vi "N-Wave Memory Generator.vi"(11 "n":i32=1) -> (0 "FXP Init Data Out":fxp<+/-,12,12>[](array[numeric]), 3 "Init Data Out":i64[](array[numeric]))   [LabVIEW 2014]
uses:
  <vilib>/Analysis/NI_AALPro.lvlib
  <vilib>/Analysis/NI_AALBase.lvlib
panel:
  out "size(s)":i32
  out "Init Data Out Graph":i64[](graph)
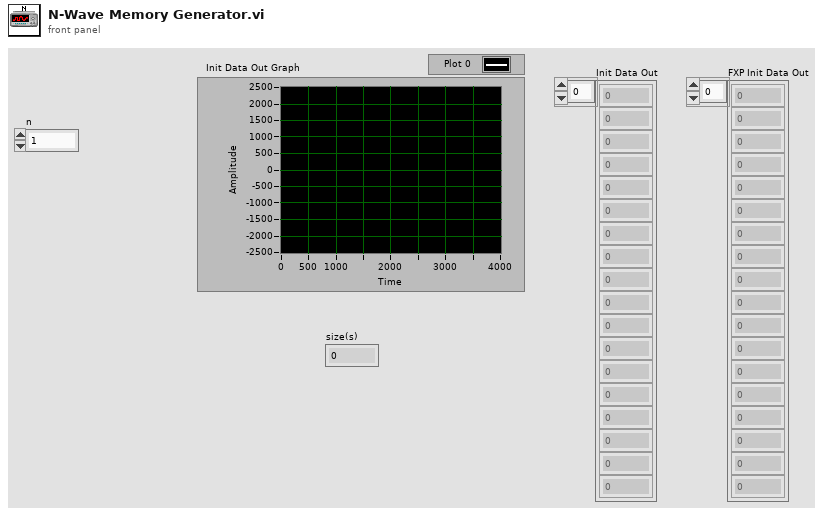
[diagram p1: front panel]
types:
  T1 = enum16{"sine", "cosine", "triangle", "square", "sawtooth", "increasing ramp", "decreasing ramp"}
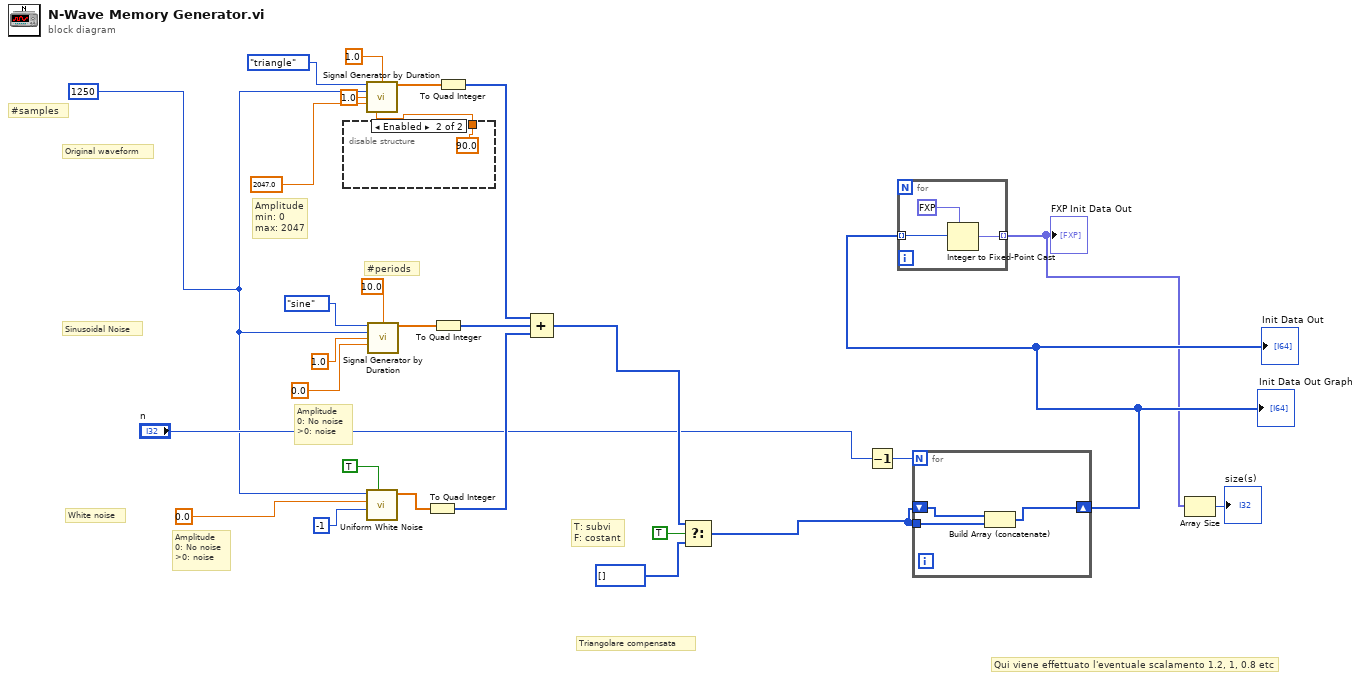
[diagram p0: block diagram]
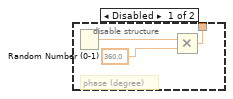
[diagram p2: hidden frame]
diagram:
  w5 = 1250 ("# of samples")
  # "Triangolare compensata"
  # "Qui viene effettuato l'eventuale scalamento 1.2, 1, 0.8 etc"
  # "T: subvi\nF: costant"
  # "Amplitude\n0: No noise\n>0: noise"
  # "Original waveform"
  # "Sinusoidal Noise"
  # "White noise"
  # "#periods"
  # "Amplitude\n0: No noise\n>0: noise"
  # "Amplitude\nmin: 0\nmax: 2047"
  # "#samples"
  n1 = disable-structure shown="Enabled" {
    disable-tunnel: [w29 90.0 ("phase in")] -> w14
    frame Disabled {
      # "phase (degree)"
      n2 = Random Number (0-1)() -> (number: 0 to 1=w30:dbl)
      n3 = Multiply(x=w30, y=360.0) -> (x*y=w29:dbl)
    }
    frame Enabled {
    }
  }
  n4 = call <vilib>:"Signal Generator by Duration.vi"("signal type"=T1."triangle", "duration"=1.0, "# of samples"=w5, "frequency"=1.0, "amplitude"=2047.0, "phase in"=w14) -> ("signal"=w16:dbl[])  [unwired: 6 in, 3 out]
  n5 = call <vilib>:"Uniform White Noise.vi"("initialize?"=TRUE, "seed"=-1, "amplitude"=0.0, "samples"=w5) -> ("uniform white noise"=w15:dbl[])  [unwired: 6 in, 1 out]
  n6 = call <vilib>:"Signal Generator by Duration.vi"("signal type"=T1."sine", "duration"=10.0, "# of samples"=w5, "frequency"=1.0, "amplitude"=0.0) -> ("signal"=w27:dbl[])  [unwired: 7 in, 3 out]
  n7 = To Quad Integer(1:w15) -> (0:w20:i64[])
  n8 = To Quad Integer(1:w27) -> (0:w22:i64[])
  n9 = To Quad Integer(1:w16) -> (0:w6:i64[])
  n10 = Compound Arithmetic op=ADD(w6, w22, w20) -> (w12:i64[])
  n11 = Select(t=w12, s=TRUE, f=i64[] []) -> (s? t:f=w11:i64[])
  n12 = Decrement(x="n") -> (x-1=w10:i32)
  n13 = for {
    N: w10 -> [_]
    shift-right: [w33] -> w3
    shift-left: w11 -> [w35]
    tunnel: w11 -> [w34]
    n14 = Build Array (concatenate)(w35, w34) -> (w33:i64[])
  }
  "Init Data Out Graph" <- w3
  "Init Data Out" <- w3
  n15 = for {
    tunnel: w3 -> [w38] mode=indexing
    tunnel: [w36] -> w1 mode=indexing
    n16 = Integer to Fixed-Point Cast(fixed-point type=fxp<+/-,12,12> 0.0, integer=w38) -> (fixed-point=w36:fxp<+/-,12,12>)
  }
  "FXP Init Data Out" <- w1
  n17 = Array Size(array=w1) -> (size(s)=→"size(s)":i32)
